vi "RT.vi"() -> ()   [LabVIEW 2017]
panel:
  in  "stop":bool
  out "Out":dbl
  in  "In":dbl
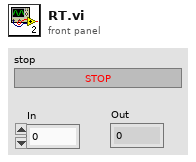
[diagram p1: front panel]
types:
  T1 = typedef "dbl.ctl" = dbl
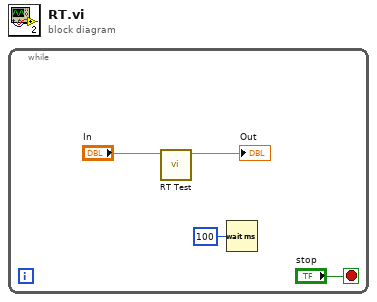
[diagram p0: block diagram]
diagram:
  n1 = while {
    stop <- "stop" stop-if-true
    n2 = call "RT Test.vi"("Data In"="In") -> ("Data Out"=→"Out":T1)  [unwired: 10 in]
    n3 = Wait (ms)(milliseconds to wait=u32 100) -> ()  [unwired: 1 out]
  }
